vi "Enum Devs.vi"() -> ()   [LabVIEW 2011, in "LVH-Adept.lvlib"]
uses:
  LVH-Adept.lvlib
  Private/DMGR/DMGR.lvlib
panel:
  out "Error Out":errorcluster
  out "Num Devices":i32
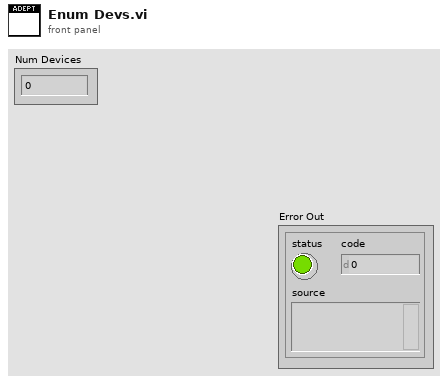
[diagram p1: front panel]
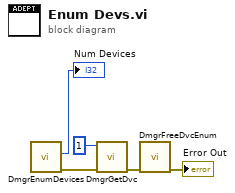
[diagram p0: block diagram]
diagram:
  n1 = call "DmgrEnumDevices.vi"() -> ("Error Out"=w4:errorcluster, "Num Devices"=→"Num Devices":i32)  [unwired: 10 in]
  n2 = call "DmgrGetDvc.vi"("Error In"=w4, "Device Number"=1) -> ("Error Out"=w3:errorcluster)  [unwired: 9 in]
  n3 = call "DmgrFreeDvcEnum.vi"("Error In"=w3) -> ("Error Out"=→"Error Out":errorcluster)  [unwired: 10 in]
